vi "Ref_Num_Set_VRMS.vi"(0 "Multiplier":refnum<vi>, 1 "Test Level Equal":refnum<vi>, 2 "Test Level value":refnum<vi>, 3 "Current LCR Voltage":refnum<vi>, 4 "TestSigLevel : current time":refnum<vi>, 5 "Test Signal Level":refnum<vi>, 6 "Signal Level : Elapsed time (seconds)":refnum<vi>, 11 "error IN":errorcluster, 12 "TestSigLevel : Started":refnum<vi>, 13 "OK Button":refnum<vi>, 14 "Stop Button":refnum<vi>) -> (8 "Error OUT":errorcluster, 10 "error Mult_0.1":errorcluster, 15 "error Mult_1":errorcluster)   [LabVIEW 2020]
uses:
  Global 1.vi
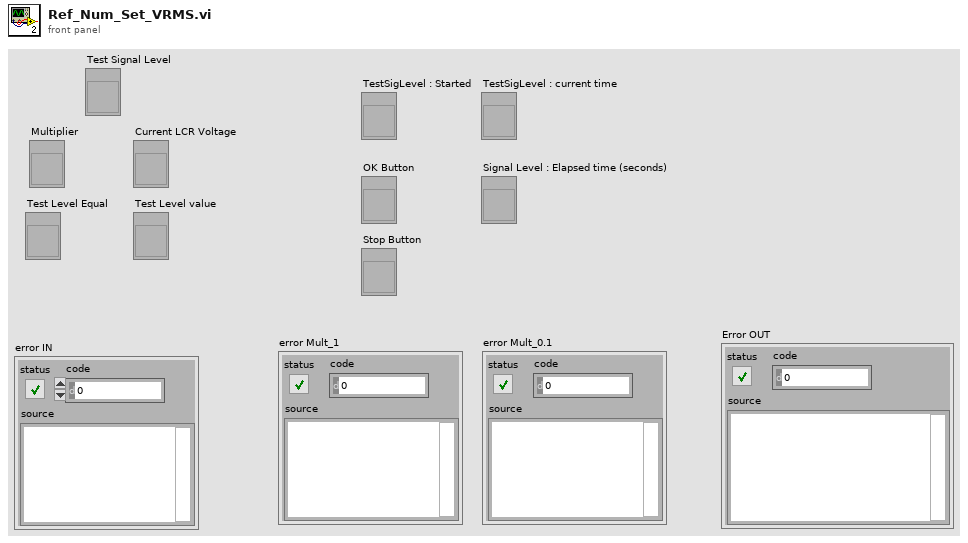
[diagram p1: front panel]
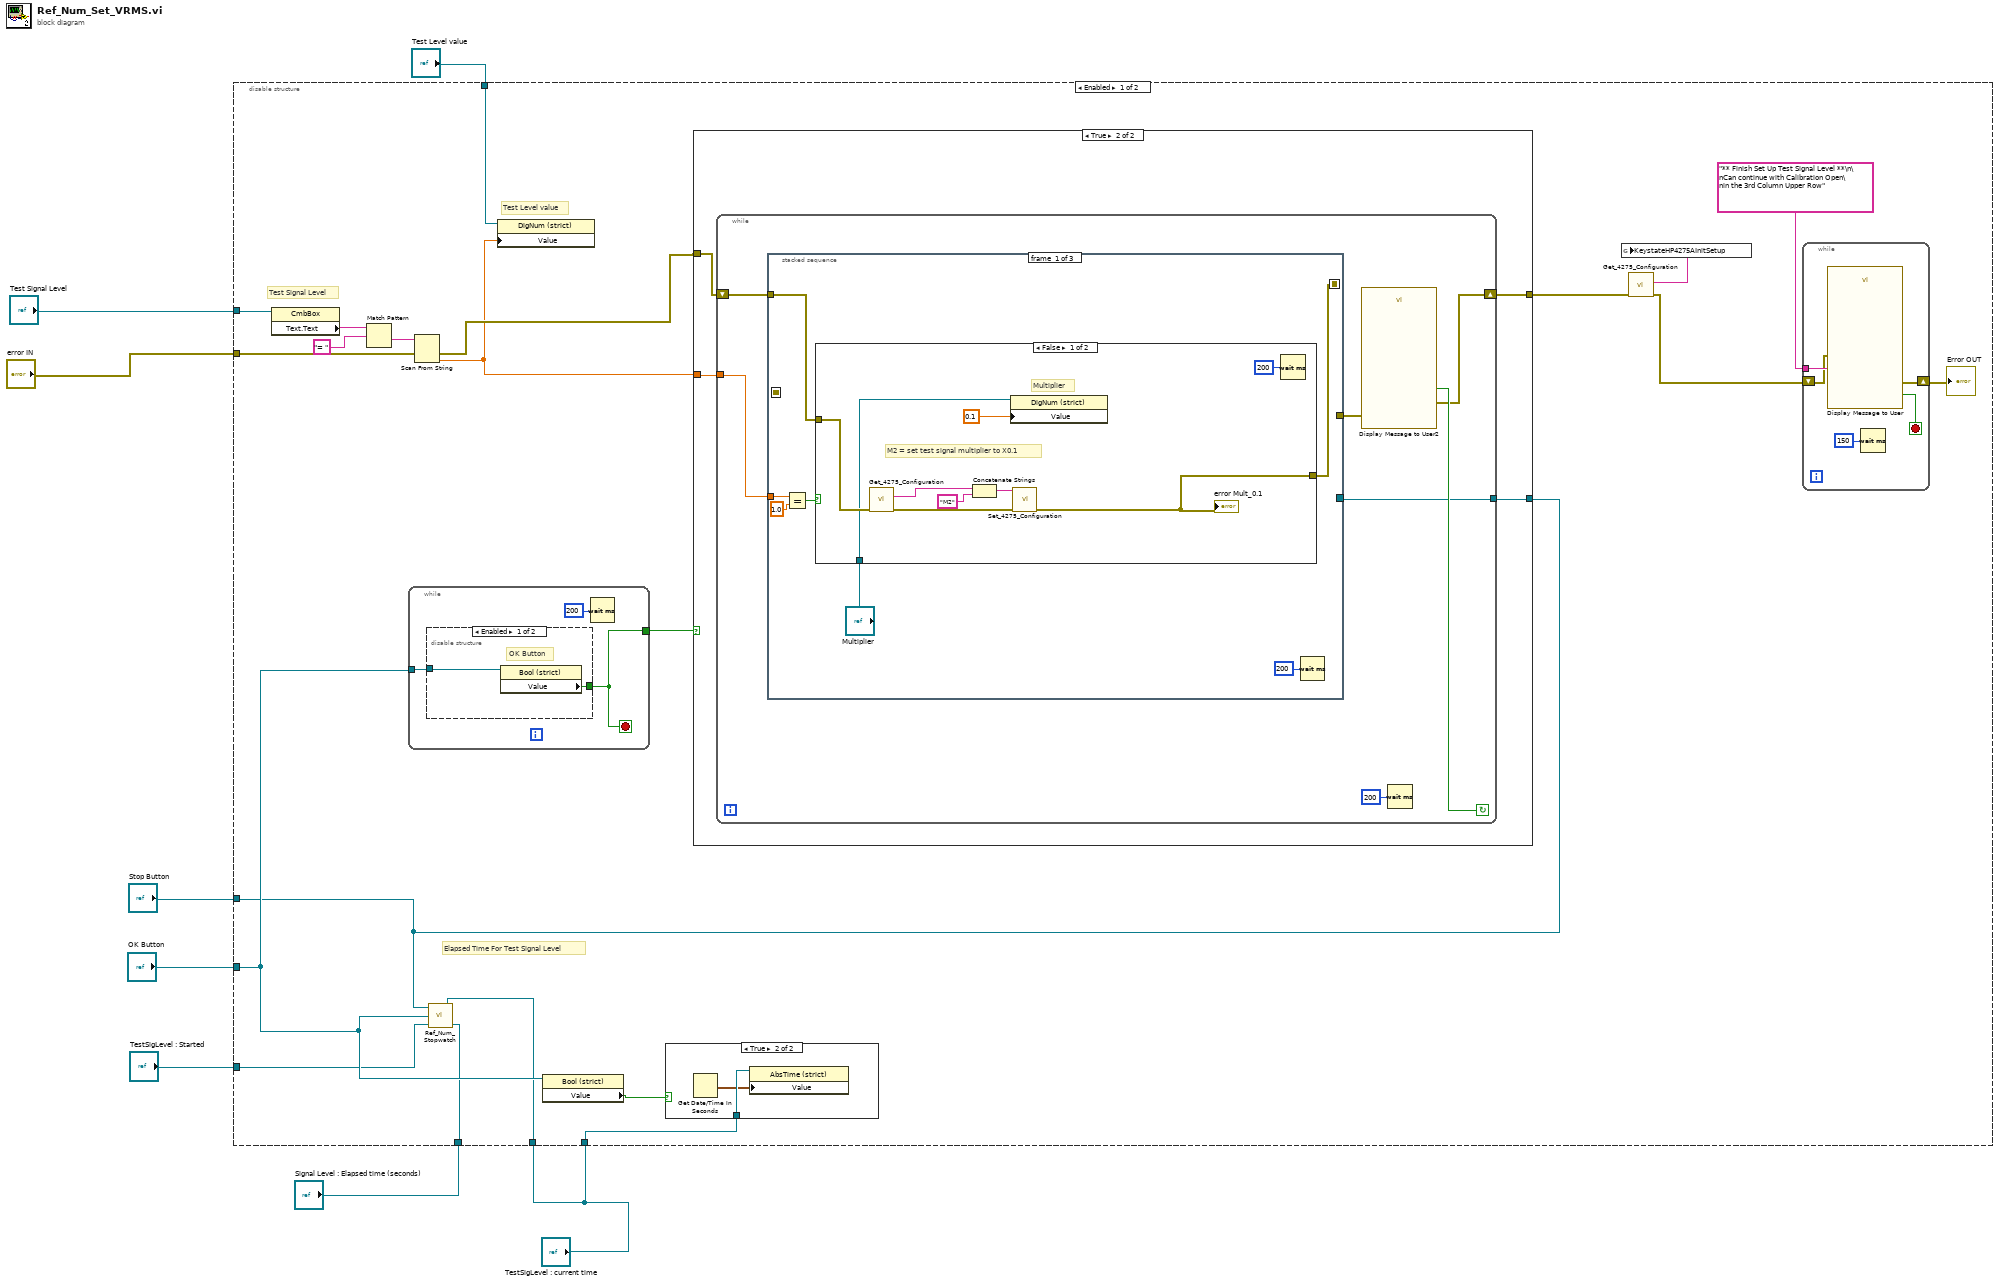
[diagram p0: block diagram]
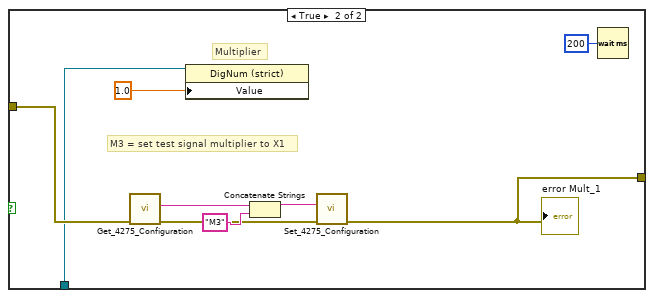
[diagram p4: hidden frame]
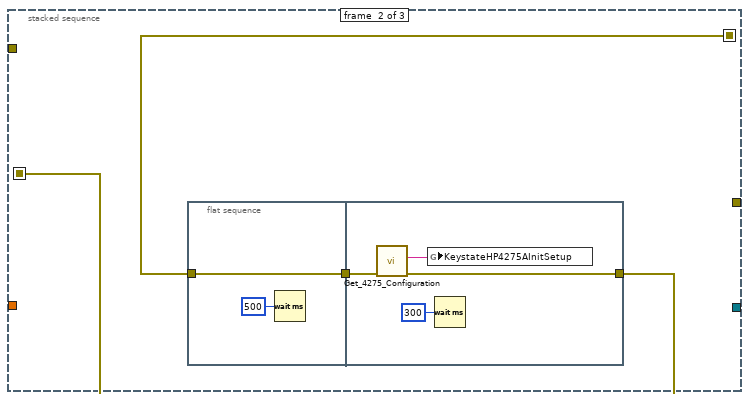
[diagram p5: hidden frame]
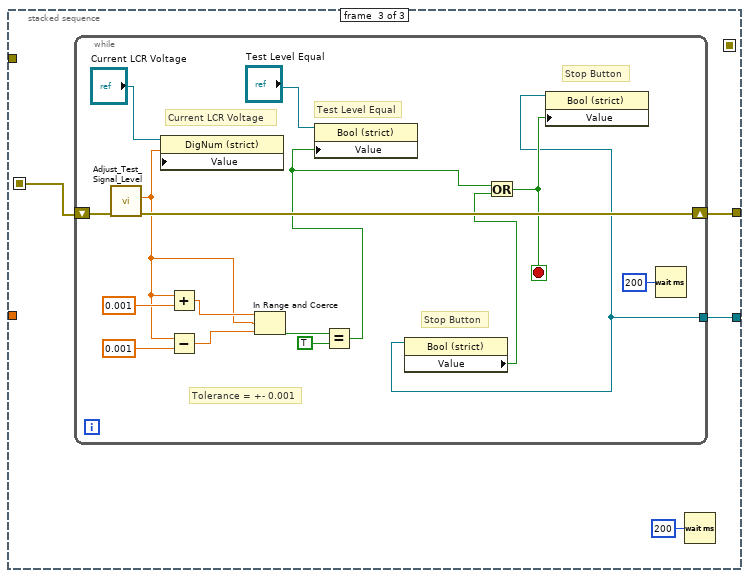
[diagram p6: hidden frame]
diagram:
  n1 = disable-structure shown="Enabled" {
    disable-tunnel: "error IN" -> [w22 _]
    disable-tunnel: "Test Signal Level" -> [w21 _]
    disable-tunnel: "Test Level value" -> [w20 _]
    disable-tunnel: "OK Button" -> [w18 _]
    disable-tunnel: "Stop Button" -> [w10 _]
    disable-tunnel: "TestSigLevel : Started" -> [w17 _]
    disable-tunnel: "Signal Level : Elapsed time (seconds)" -> [w16 _]
    disable-tunnel: "TestSigLevel : current time" -> [w15 _]
    disable-tunnel: "TestSigLevel : current time" -> [w14 _]
    frame Enabled {
      # "Test Signal Level"
      # "Test Level value"
      # "Elapsed Time For Test Signal Level"
      n2 = property on="Property Node" class="CmbBox"(reference=w21) -> ("Text.Text"=w29:string)  [unwired: 1 in, 2 out]
      n3 = Match Pattern(string=w29, regular expression="= ") -> (after substring=w27:string)  [unwired: 1 in, 3 out]
      n4 = while {
        tunnel: [w36] -> w24
        tunnel: w18 -> [w37]
        stop <- w36 stop-if-true
        n5 = disable-structure shown="Enabled" {
          disable-tunnel: [w39 _] -> w36
          disable-tunnel: w37 -> [w38 _]
          frame Enabled {
            # "OK Button"
            n6 = property class="Bool (strict)"(reference=w38) -> ("Value"=w39:bool)  [unwired: 1 in, 2 out]
          }
          frame Disabled {
          }
        }
        n7 = Wait (ms)(milliseconds to wait=u32 200) -> ()  [unwired: 1 out]
      }
      n8 = Scan From String(input string=w27, error in=w22) -> (error out=w23:errorcluster, output 1=w19:dbl)  [unwired: 3 in, 2 out]
      n9 = call "Ref_Num_Stopwatch.vi"("Elapsed time (seconds)"=w16, "start time"=w15, "Started"=w17, "OK Button"=w18, "stop"=w10) -> ()  [unwired: 1 in]
      n10 = property class="DigNum (strict)"(reference=w20, "Value"=w19) -> ()  [unwired: 1 in, 2 out]
      n11 = property class="Bool (strict)"(reference=w18) -> ("Value"=w25:bool)  [unwired: 1 in, 2 out]
      n12 = case shown="True" w25 {
        tunnel: w14 -> [_ w107]
        frame False {
        }
        frame True {
          n13 = Get Date/Time In Seconds() -> (seconds since 1Jan1904=w106:timestamp)
          n14 = property class="AbsTime (strict)"(reference=w107, "Value"=w106) -> ()  [unwired: 1 in, 2 out]
        }
      }
      n15 = case shown="True" w24 {
        tunnel: w23 -> [w40 w43]
        tunnel: w19 -> [_ w44]
        tunnel: [w40 w42] -> w12
        tunnel: w10 -> [_ w41]
        frame False {
        }
        frame True {
          n16 = while {
            tunnel: w44 -> [w47]
            tunnel: w41 -> [w45]
            shift-right: [w49] -> w42
            shift-left: w43 -> [w46]
            stop <- w51 continue-if-true
            n17 = stacked-sequence {
              seq-local: [w53 _ _] -> [_ w79 _]
              seq-local: [_ w77 _] -> [_ _ w86]
              tunnel: w45 -> [_ _ w89]
              tunnel: [_ _ w88] -> w50
              tunnel: w47 -> [w57 _ _]
              tunnel: w46 -> [w55 _ _]
              frame #0 {
                n18 = Equal?(x=w57, y=1.0) -> (x = y?=w56:bool)
                n19 = case shown="False" w56 {
                  tunnel: w55 -> [w64 w72]
                  tunnel: [w59 w68] -> w53
                  tunnel: "Multiplier" -> [w60 w69]
                  frame False {
                    # "Multiplier"
                    # "M2 = set test signal multiplier to X0.1"
                    n20 = call "Get_4275_Configuration.vi"("error in"=w64) -> ("error out"=w63:errorcluster, "Keystate"=w66:string)  [unwired: 9 in]
                    n21 = Concatenate Strings(w66, "M2" ("string")) -> (w65:string)
                    n22 = property class="DigNum (strict)"(reference=w60, "Value"=0.1) -> ()  [unwired: 1 in, 2 out]
                    n23 = call "Set_4275_Configuration.vi"("error in"=w63, "Keystate"=w65) -> ("error out"=w59:errorcluster)  [unwired: 9 in]
                    "error Mult_0.1" <- w59
                    n24 = Wait (ms)(milliseconds to wait=u32 200) -> ()  [unwired: 1 out]
                  }
                  frame True {
                    # "Multiplier"
                    # "M3 = set test signal multiplier to X1"
                    n25 = call "Get_4275_Configuration.vi"("error in"=w72) -> ("error out"=w73:errorcluster, "Keystate"=w76:string)  [unwired: 9 in]
                    n26 = property class="DigNum (strict)"(reference=w69, "Value"=1.0 ("Multiplier")) -> ()  [unwired: 1 in, 2 out]
                    n27 = Concatenate Strings(w76, "M3" ("string")) -> (w74:string)
                    n28 = call "Set_4275_Configuration.vi"("error in"=w73, "Keystate"=w74) -> ("error out"=w68:errorcluster)  [unwired: 9 in]
                    "error Mult_1" <- w68
                    n29 = Wait (ms)(milliseconds to wait=u32 200) -> ()  [unwired: 1 out]
                  }
                }
                n30 = Wait (ms)(milliseconds to wait=u32 200) -> ()  [unwired: 1 out]
              }
              frame #1 {
                n31 = flat-sequence {
                  tunnel: w79 -> [w81]
                  tunnel: [w81] -> w78
                  tunnel: w78 -> [w84]
                  tunnel: [w83] -> w77
                  frame #0 {
                    n32 = Wait (ms)(milliseconds to wait=u32 500) -> ()  [unwired: 1 out]
                  }
                  frame #1 {
                    n33 = call "Get_4275_Configuration.vi"("error in"=w84) -> ("error out"=w83:errorcluster, "Keystate"=w85:string)  [unwired: 9 in]
                    n34 = global write "Global 1.vi" "KeystateHP4275AInitSetup"(w85) -> ()
                    n35 = Wait (ms)(milliseconds to wait=u32 300) -> ()  [unwired: 1 out]
                  }
                }
              }
              frame #2 {
                n36 = while {
                  tunnel: w89 -> [w92]
                  shift-right: [w104] -> w88
                  shift-left: w86 -> [w105]
                  stop <- w94 stop-if-true
                  # "Stop Button"
                  # "Stop Button"
                  # "Test Level Equal"
                  # "Current LCR Voltage"
                  # "Tolerance = +- 0.001"
                  n37 = call "Adjust_Test_Signal_Level.vi"("error in"=w105) -> ("error out"=w104:errorcluster, "OscVoltage"=w96:dbl)  [unwired: 9 in]
                  n38 = property class="DigNum (strict)"(reference="Current LCR Voltage", "Value"=w96) -> ()  [unwired: 1 in, 2 out]
                  n39 = Add(x=w96, y=0.001) -> (x+y=w100:dbl)
                  n40 = Subtract(x=w96, y=0.001) -> (x-y=w99:dbl)
                  n41 = In Range and Coerce(upper limit=w100, x=w96, lower limit=w99) -> (In Range?=w98:bool)  [unwired: 1 out]
                  n42 = Equal?(x=w98, y=TRUE) -> (x = y?=w95:bool)
                  n43 = property class="Bool (strict)"(reference="Test Level Equal", "Value"=w95) -> ()  [unwired: 1 in, 2 out]
                  n44 = property class="Bool (strict)"(reference=w92) -> ("Value"=w93:bool)  [unwired: 1 in, 2 out]
                  n45 = Or(x=w95, y=w93) -> (x .or. y?=w94:bool)
                  n46 = property class="Bool (strict)"(reference=w92, "Value"=w94) -> ()  [unwired: 1 in, 2 out]
                  n47 = Wait (ms)(milliseconds to wait=u32 200) -> ()  [unwired: 1 out]
                }
                n48 = Wait (ms)(milliseconds to wait=u32 200) -> ()  [unwired: 1 out]
              }
            }
            n49 = call "Display Message to User2"("error in (no error)"=w50) -> ("error out"=w49:errorcluster, "NO"=w51:bool)  [unwired: 9 in]
            n50 = Wait (ms)(milliseconds to wait=u32 200) -> ()  [unwired: 1 out]
          }
        }
      }
      n51 = call "Get_4275_Configuration.vi"("error in"=w12) -> ("error out"=w11:errorcluster, "Keystate"=w13:string)  [unwired: 9 in]
      n52 = global write "Global 1.vi" "KeystateHP4275AInitSetup"(w13) -> ()
      n53 = while {
        tunnel: "** Finish Set Up Test Signal Level **\n\nCan continue with Calibration Open\nin the 3rd Column Upper Row" ("message") -> [w34]
        shift-right: [w31] -> w9
        shift-left: w11 -> [w33]
        stop <- w32 stop-if-true
        n54 = call "Display Message to User"("error in (no error)"=w33, "Message"=w34) -> ("error out"=w31:errorcluster, "OK"=w32:bool)  [unwired: 8 in]
        n55 = Wait (ms)(milliseconds to wait=u32 150) -> ()  [unwired: 1 out]
      }
      "Error OUT" <- w9
    }
    frame Disabled {
    }
  }
